vi "Get FIFO Flags.vi"(11 "Debug Flags in":refnum<class "Debug Flags.lvclass">) -> (2 "FIFO":refnum<class "Debug Flags FIFO.lvclass">, 3 "Debug Flags out":refnum<class "Debug Flags.lvclass">)   [LabVIEW 2017, in "Data Sharing Framework Engine.lvlib" / "Debug Flags.lvclass"]
uses:
  Debug Flags.lvclass
  Debug Flags FIFO/Debug Flags FIFO.lvclass
  Debug Flags.lvclass/Debug Flags.ctl
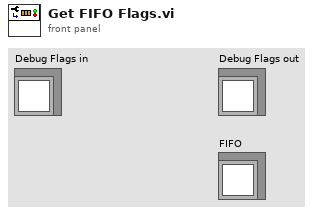
[diagram p1: front panel]
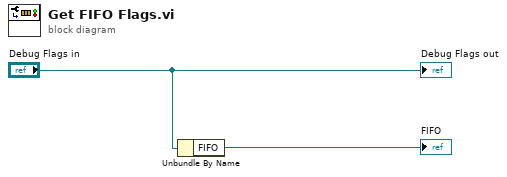
[diagram p0: block diagram]
diagram:
  n1 = Unbundle By Name("Debug Flags in") -> ("FIFO"=→"FIFO":refnum<class "Debug Flags FIFO.lvclass">)
  "Debug Flags out" <- "Debug Flags in"
